vi "getAllClasses.vi"(8 "error in":errorcluster) -> (0 "error out":errorcluster, 2 "all classes":string[](array[string]))   [LabVIEW 2020, in "JKI JSON Object Serialization.lvlib" / "OOP_Utility.lvlib" / "Reflection.lvclass"]
doc: "Get the class hierarchy for the specified class. The first element of the output array is the top most parent class; the last element is the input class. Input className can include or exclude the '.lvclass' extension. Output values include '.lvclass' extension.\n\nGCraftsman JSON Object Serialization Toolkit\nwww.GCraftsman.com\nCopyright (c) 2017, GCraftsman"
uses:
  Reflection.lvclass
  reflectionPoolAction.ctl
  Reflection.lvclass/Reflection.ctl
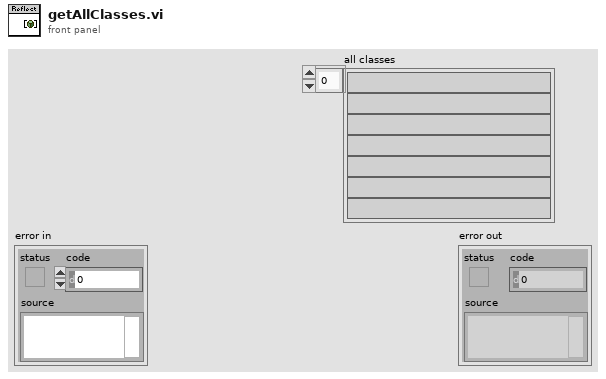
[diagram p1: front panel]
types:
  T1 = typedef "JKI JSON Object Serialization.lvlib/OOP_Utility.lvlib/Reflection.lvclass/reflectionPoolAction.ctl" = enum16{"<select>", "getPrivateData", "getClassHierarchy", "getClassVersions", "getAllClasses"}
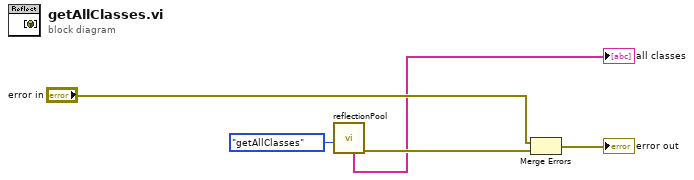
[diagram p0: block diagram]
diagram:
  n1 = call "reflectionPool.vi"("action"=reflectionPoolAction."getAllClasses") -> ("error out"=w3:errorcluster, "allClassNames"=→"all classes":string[])  [unwired: 5 in, 4 out]
  n2 = Merge Errors("error in", w3) -> (→"error out":errorcluster)
